vi "VI-Create XControl Property.vi"(0 "Path":path=path "C:/Users/hancock/Desktop/Test/Test.xctl", 5 "Name":string="NewProp", 7 "Direction":u16(ring) items=["Read/Write", "Read only", "Write only"], 9 "Data Type In":variant, 11 "error in (no error)":errorcluster, 12 "Where":i32) -> (15 "error out":errorcluster)   [LabVIEW 2015]
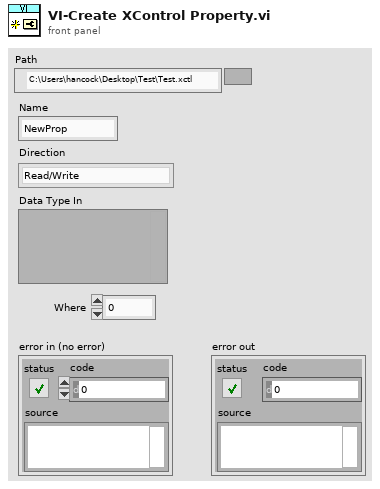
[diagram p1: front panel]
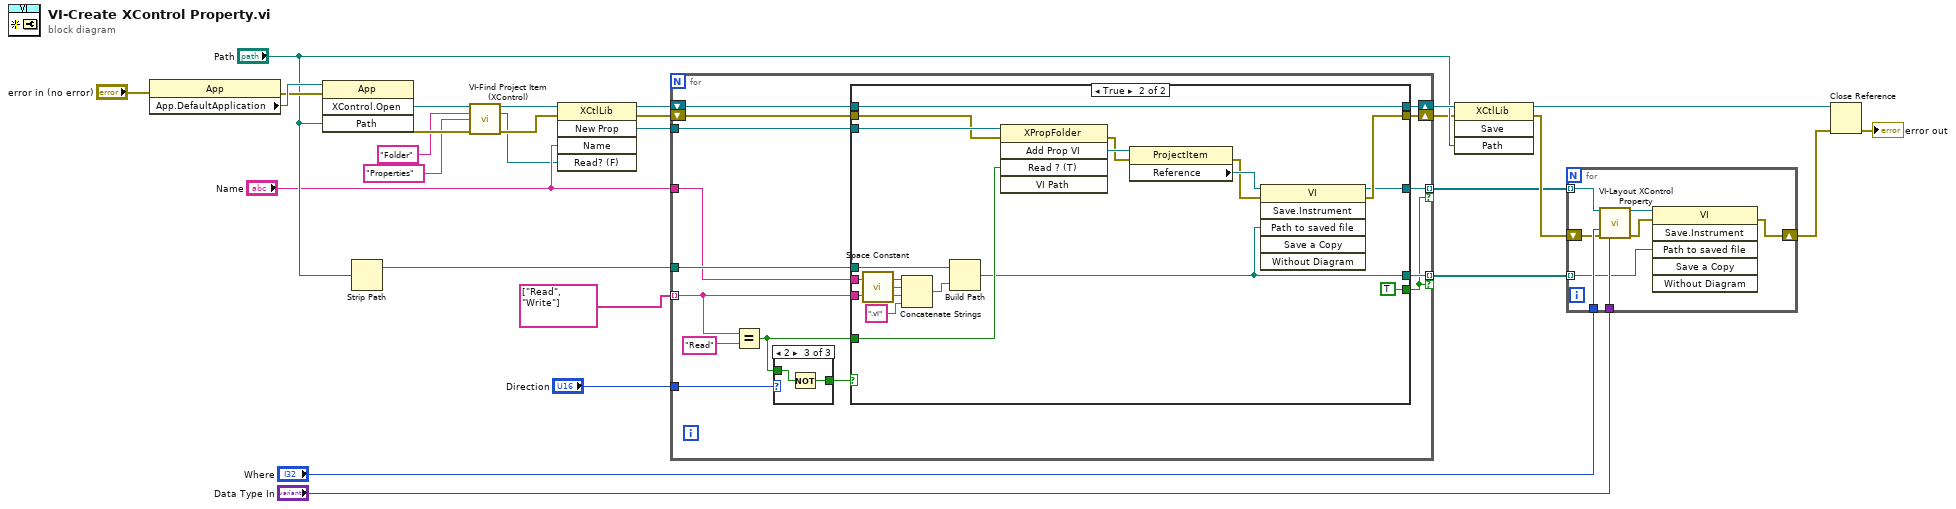
[diagram p0: block diagram]
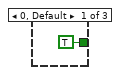
[diagram p2: hidden frame]
diagram:
  n1 = property class="App"(error in="error in (no error)") -> (error out=w23:errorcluster, "App.DefaultApplication"=w24:refnum<vi>)  [unwired: 1 in, 1 out]
  n2 = invoke class="App" method="XControl.Open"(reference=w24, error in=w23, "Path"="Path") -> (error out=w26:errorcluster, "Open XControl"=w27:refnum<vi>)  [unwired: 1 in, 2 out]
  n3 = Strip Path(path="Path") -> (stripped path=w25:path)  [unwired: 1 out]
  n4 = call "VI-Find Project Item (XControl).vi"("XCtlLib Refnum"=w27, "Type"="Folder" ("y"), "Name"="Properties" ("y"), "error in (no error)"=w26) -> ("reference out"=w21:refnum<vi>, "ProjectItem"=w11:refnum<vi>, "error out"=w14:errorcluster)  [unwired: 9 in]
  n5 = invoke class="XCtlLib" method="New Prop"(reference=w21, error in=w14, "Name"="Name", "Read? (F)"=w11) -> (reference out=w15:refnum<vi>, error out=w13:errorcluster, "New Prop"=w10:refnum<vi>)  [unwired: 1 in, 2 out]
  n6 = for {
    tunnel: w25 -> [w41]
    tunnel: "Name" -> [w32]
    tunnel: string[] ["Read", "Write"] ("string") -> [w40] mode=indexing
    shift-right: [w43] -> w22
    shift-left: w15 -> [w35]
    shift-right: [w42] -> w6
    shift-left: w13 -> [w34]
    tunnel: "Direction" -> [w38]
    tunnel: w10 -> [w33]
    tunnel: [w31] -> w8 mode=indexing if=w29
    tunnel: [w30] -> w3 mode=indexing if=w29
    n7 = Equal?(x=w40, y="Read") -> (x = y?=w37:bool)
    n8 = case shown="2" w38 {
      tunnel: w37 -> [_ w45 w47]
      tunnel: [TRUE w45 w46] -> w36
      frame 0, Default {
      }
      frame 1 {
      }
      frame 2 {
        n9 = Not(x=w47) -> (.not. x?=w46:bool)
      }
    }
    n10 = case shown="True" w36 {
      tunnel: [w49 w56] -> w43
      tunnel: w35 -> [w49 w56]
      tunnel: [w48 w60] -> w42
      tunnel: w34 -> [w48 w57]
      tunnel: w41 -> [_ w66]
      tunnel: w40 -> [_ w64]
      tunnel: w37 -> [_ w61]
      tunnel: w33 -> [_ w59]
      tunnel: w32 -> [_ w58]
      tunnel: [_ w52] -> w31
      tunnel: [_ TRUE] -> w29
      tunnel: [_ w50] -> w30
      frame False {
      }
      frame True {
        n11 = call <vilib>:"Space Constant.vi"() -> ("String"=w62:string)
        n12 = Concatenate Strings(w58, w62, w64, ".vi" ("string")) -> (w65:string)
        n13 = Build Path(base path=w66, name or relative path=w65) -> (appended path=w52:path)
        n14 = invoke class="XPropFolder" method="Add Prop VI"(reference=w59, error in=w57, "Read ? (T)"=w61) -> (error out=w55:errorcluster, "Add Prop VI"=w67:refnum<vi>)  [unwired: 2 in, 3 out]
        n15 = property class="ProjectItem"(reference=w67, error in=w55) -> (error out=w53:errorcluster, "Reference"=w54:refnum<vi>)  [unwired: 1 out]
        n16 = invoke class="VI" method="Save.Instrument"(reference=w54, error in=w53, "Path to saved file"=w52) -> (reference out=w50:refnum<vi>, error out=w60:errorcluster)  [unwired: 3 in, 4 out]
      }
    }
  }
  n17 = invoke class="XCtlLib" method="Save"(reference=w22, error in=w6, "Path"="Path") -> (reference out=w9:refnum<vi>, error out=w4:errorcluster)  [unwired: 1 in, 2 out]
  n18 = for {
    tunnel: w8 -> [w70] mode=indexing
    tunnel: "Data Type In" -> [w75]
    tunnel: "Where" -> [w74]
    tunnel: w3 -> [w73] mode=indexing
    shift-right: [w68] -> w2
    shift-left: w4 -> [w72]
    n19 = call "VI-Layout XControl Property.vi"("VI in"=w73, "Where"=w74, "error in (no error)"=w72, "Data Type In"=w75) -> ("VI out"=w71:refnum<vi>, "error out"=w69:errorcluster)  [unwired: 9 in, 1 out]
    n20 = invoke class="VI" method="Save.Instrument"(reference=w71, error in=w69, "Path to saved file"=w70) -> (error out=w68:errorcluster)  [unwired: 3 in, 5 out]
  }
  n21 = Close Reference(reference=w9, error in (no error)=w2) -> (error out=→"error out":errorcluster)
